vi "isconnect.vi"(0 "duplicate VISA resource name":refnum<visa-resource-name>, 1 "error in":errorcluster) -> (2 "dup VISA resource name":refnum<visa-resource-name>, 3 "Boolean":bool, 4 "error out":errorcluster)   [LabVIEW 2010]
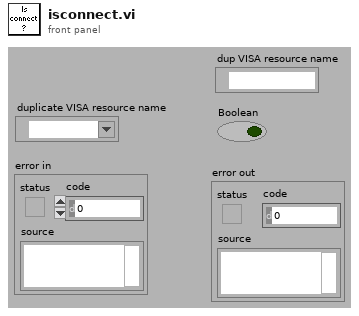
[diagram p1: front panel]
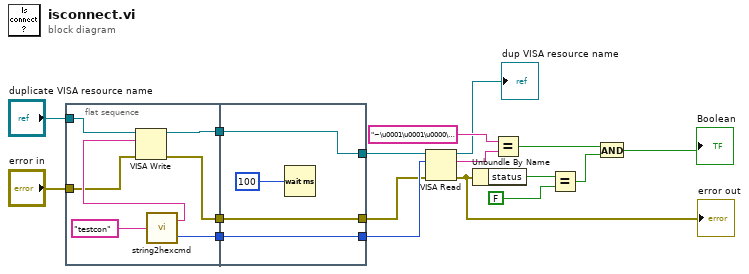
[diagram p0: block diagram]
diagram:
  n1 = flat-sequence {
    tunnel: "duplicate VISA resource name" -> [w21]
    tunnel: "error in" -> [w19]
    tunnel: [w24] -> w3
    tunnel: [w23] -> w2
    tunnel: [w18] -> w1
    tunnel: [w26] -> w4
    tunnel: [w27] -> w8
    tunnel: [w28] -> w9
    tunnel: w3 -> [w28]
    tunnel: w2 -> [w27]
    tunnel: w1 -> [w26]
    frame #0 {
      n2 = call "string2hexcmd.vi"("String comand"="testcon") -> ("hex comand"=w22:string, "byte count"=w24:u32)
      n3 = VISA Write(VISA resource name=w21, write buffer=w22, error in (no error)=w19) -> (VISA resource name out=w23:refnum<visa-resource-name>, error out=w18:errorcluster)  [unwired: 1 out]
    }
    frame #1 {
      n4 = Wait (ms)(milliseconds to wait=100) -> ()  [unwired: 1 out]
    }
  }
  n5 = VISA Read(VISA resource name=w8, byte count=w9, error in (no error)=w4) -> (VISA resource name out=→"dup VISA resource name":refnum<visa-resource-name>, read buffer=w11:string, error out=w17:errorcluster)  [unwired: 1 out]
  "error out" <- w17
  n6 = Unbundle By Name(w17) -> ("status"=w12:bool)
  n7 = Equal?(x="~\u0001\u0001\u0000\u0000\u0000", y=w11) -> (x = y?=w13:bool)
  n8 = Equal?(x=w12, y=FALSE) -> (x = y?=w14:bool)
  n9 = And(x=w13, y=w14) -> (x .and. y?=→"Boolean":bool)
